vi "Event Create.vi"(9 "Event jettl":refnum<class "Event jettl.lvclass">, 10 "Alias":string, 11 "Base Queue jettl in":refnum<class "Base Queue jettl.lvclass">) -> (3 "Base Queue jettl out":refnum<class "Base Queue jettl.lvclass">)   [LabVIEW 2021, in "jettl.lvlib" / "Base Queue jettl.lvlib" / "Base Queue jettl.lvclass"]
uses:
  Base Queue jettl.lvclass
  Event jettl/Event jettl.lvclass
  Msg Strategy/Msg Strategy.lvclass
  Base Queue jettl.lvclass/Base Queue jettl.ctl
  jettl.lvlib
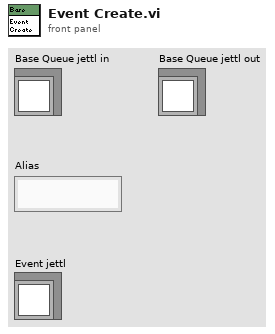
[diagram p1: front panel]
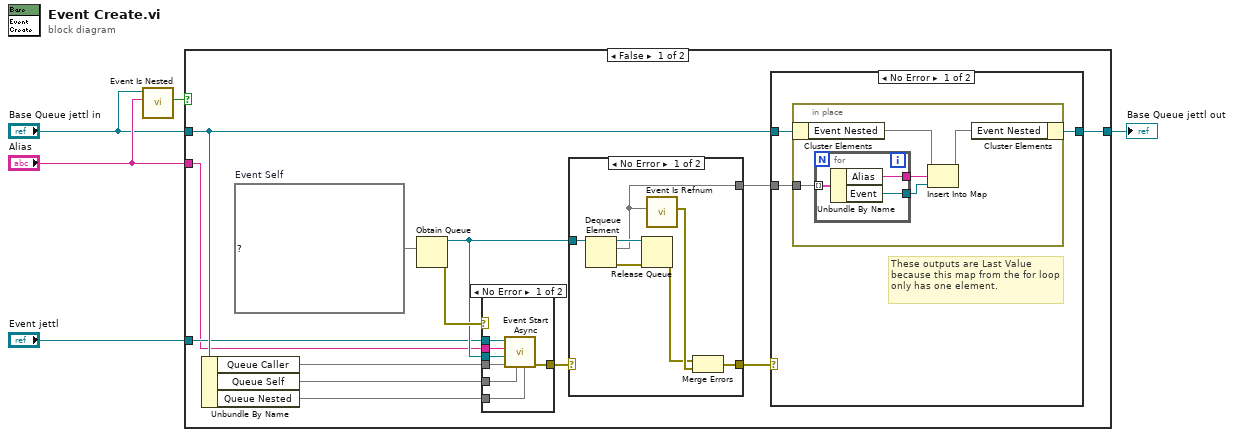
[diagram p0: block diagram]
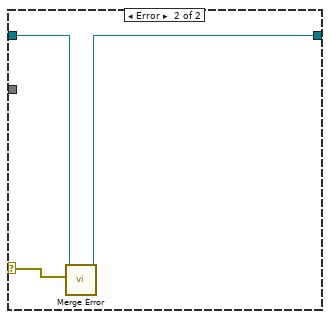
[diagram p4: hidden frame]
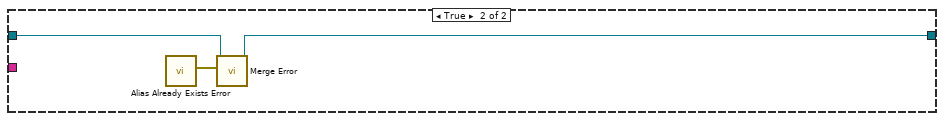
[diagram p5: hidden frame]
diagram:
  n1 = call-dynamic "Event Is Nested.vi"("Alias"="Alias", "Base Queue jettl in"="Base Queue jettl in") -> ("Event Is Nested?"=w3:bool)  [unwired: 9 in]
  n2 = case shown="False" w3 {
    tunnel: "Event jettl" -> [w13 _]
    tunnel: "Base Queue jettl in" -> [w16 w51]
    tunnel: "Alias" -> [w12 _]
    tunnel: [w15 w50] -> w4
    frame False {
      w11 = map{string, refnum<data-value>} {}  # Event Self
      n3 = Unbundle By Name(w16) -> ("Queue Caller"=w8:map{string, refnum<data-value>}, "Queue Self"=w7:map{string, refnum<data-value>}, "Queue Nested"=w6:map{string, refnum<data-value>})
      n4 = Obtain Queue(element data type=w11) -> (queue out=w14:refnum<queue>, error out=w18:errorcluster)  [unwired: 4 in, 1 out]
      n5 = case shown="No Error" w18 {
        selector: w18 -> [_ w34]
        tunnel: [w30 w34] -> w9
        tunnel: w13 -> [w33 _]
        tunnel: w14 -> [w31 _]
        tunnel: w12 -> [w32 _]
        tunnel: w8 -> [w29 _]
        tunnel: w7 -> [w28 _]
        tunnel: w6 -> [w27 _]
        frame No Error {
          n6 = call "Event Start Async.vi"("Queue Nested"=w27, "Queue Self"=w28, "Queue Caller"=w29, "Queue of Event Self"=w31, "Event Self Alias"=w32, "Event jettl"=w33) -> ("error out"=w30:errorcluster)  [unwired: 5 in]
        }
        frame Error {
        }
      }
      n7 = case shown="No Error" w9 {
        selector: w9 -> [_ w26]
        tunnel: [w23 w26] -> w17
        tunnel: w14 -> [w22 _]
        tunnel: [w21 _] -> w10
        frame No Error {
          n8 = Dequeue Element(queue=w22) -> (queue out=w24:refnum<queue>, element=w21:map{string, refnum<data-value>}, error out=w25:errorcluster)  [unwired: 2 in, 1 out]
          n9 = Release Queue(queue=w24, error in (no error)=w25) -> (error out=w19:errorcluster)  [unwired: 1 in, 2 out]
          n10 = call "Event Is Refnum.vi"("Event Self"=w21) -> ("Error"=w20:errorcluster)  [unwired: 10 in]
          n11 = Merge Errors(w19, w20) -> (w23:errorcluster)
        }
        frame Error {
        }
      }
      n12 = case shown="No Error" w17 {
        selector: w17 -> [_ w46]
        tunnel: w16 -> [w37 w48]
        tunnel: [w36 w47] -> w15
        tunnel: w10 -> [w35 _]
        frame No Error {
          # "These outputs are Last Value because this map from the for loop only has one element."
          n13 = in-place {
            in-place-border: w35 -> [w40]
            n14 = in-place-cluster #1(w37) -> ("Event Nested"=w42:map{string, refnum<data-value>})
            n15 = for {
              tunnel: w40 -> [w45] mode=indexing
              tunnel: [w44] -> w39
              tunnel: [w43] -> w38
              n16 = Unbundle By Name(w45) -> ("Alias"=w44:string, "Event"=w43:refnum<data-value>)
            }
            n17 = Insert Into Map(map in=w42, key=w39, value=w38) -> (map out=w41:map{string, refnum<data-value>})  [unwired: 2 out]
            n18 = in-place-cluster #1("Event Nested"=w41) -> (w36:refnum<class "Base Queue jettl.lvclass">)
          }
        }
        frame Error {
          n19 = call-dynamic "Merge Error.vi"("Error"=w46, "Base Queue jettl in"=w48) -> ("Base Queue jettl out"=w47:refnum<class "Base Queue jettl.lvclass">)  [unwired: 9 in]
        }
      }
    }
    frame True {
      n20 = call "Alias Already Exists Error.vi"() -> ("Error"=w49:errorcluster)  [unwired: 11 in]
      n21 = call-dynamic "Merge Error.vi"("Error"=w49, "Base Queue jettl in"=w51) -> ("Base Queue jettl out"=w50:refnum<class "Base Queue jettl.lvclass">)  [unwired: 9 in]
    }
  }
  "Base Queue jettl out" <- w4
